vi "ErrorText.vi"(11 "ErrNo":i32) -> (2 "Error":bool, 3 "ErrMessage":string)   [LabVIEW 2020, in "SnapMB.lvlib"]
uses:
  SnapMB.lvlib
  windows/snapmb.dll
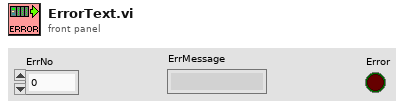
[diagram p1: front panel]
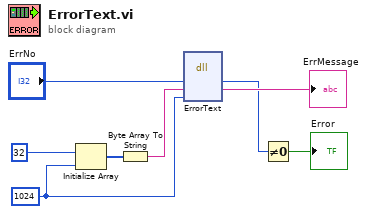
[diagram p0: block diagram]
diagram:
  w4 = 1024 ("Dimension Size")
  n1 = Initialize Array(u8 32 ("Element Data"), w4) -> (w6:u8[])
  n2 = Byte Array To String(unsigned byte array=w6) -> (string=w7:string)
  n3 = dll-call lib="D:/SnapMB/LabView/lib/windows/snapmb.dll" fn="ErrorText"("Error"="ErrNo", "ErrMessage"=w7, "TextLen"=w4) -> ("Error"=w1:i32, "ErrMessage"=→"ErrMessage":string)  [unwired: 5 in, 2 out]
  n4 = Not Equal To 0?(x=w1) -> (x != 0?=→"Error":bool)
